vi "Move To Chuck.vi"(7 "Move if Same":bool=TRUE, 8 "error in":errorcluster, 9 "Speed(mm/s)":dbl=50.0, 10 "Chuck":i32, 11 "Gantry in":refnum<class "Gantry Class.lvclass">) -> (0 "error out":errorcluster, 3 "Gantry out":refnum<class "Gantry Class.lvclass">)   [LabVIEW 2011, in "Gantry Class.lvclass"]
uses:
  Gantry Class.lvclass
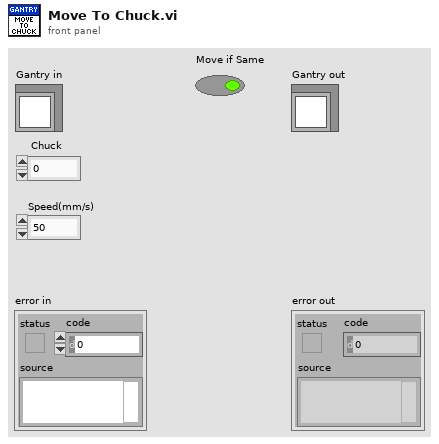
[diagram p1: front panel]
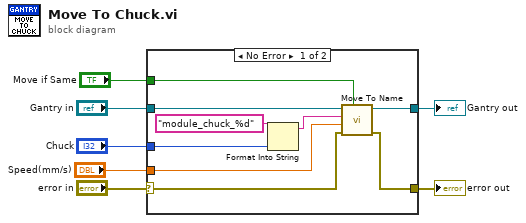
[diagram p0: block diagram]
diagram:
  n1 = case shown="No Error" "error in" {
    selector: "error in" -> [w9 w18]
    tunnel: [w8 w18] -> w6
    tunnel: [w10 w17] -> w4
    tunnel: "Gantry in" -> [w13 w17]
    tunnel: "Chuck" -> [w16 _]
    tunnel: "Move if Same" -> [w12 _]
    tunnel: "Speed(mm/s)" -> [w11 _]
    frame No Error {
      n2 = Format Into String(format string="module_chuck_%d", w16) -> (resulting string=w14:string)  [unwired: 2 in, 1 out]
      n3 = call-dynamic "Move To Name.vi"("Move if Same"=w12, "error in"=w9, "Speed(mm/s)"=w11, "Destination Name"=w14, "Gantry in"=w13) -> ("error out"=w8:errorcluster, "Gantry out"=w10:refnum<class "Gantry Class.lvclass">)  [unwired: 5 in]
    }
    frame Error {
    }
  }
  "error out" <- w6
  "Gantry out" <- w4
